vi "PropertyObjectFile Ref.vi"(8 "error in (no error)":errorcluster, 11 "PropertyObjectFile in":refnum<class "PropertyObjectFile.lvclass">) -> (0 "error out":errorcluster, 2 "PropertyObjectFile":refnum<k7>, 3 "PropertyObjectFile out":refnum<class "PropertyObjectFile.lvclass">)   [LabVIEW 2020, in "TSnax.lvlib" / "PropertyObjectFile.lvclass"]
uses:
  PropertyObjectFile.lvclass
  PropertyObjectFile.lvclass/PropertyObjectFile.ctl
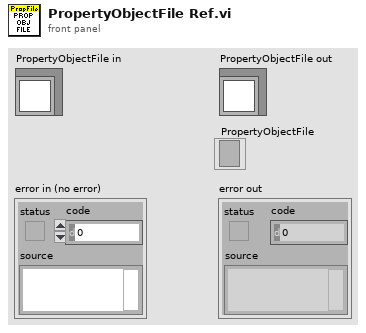
[diagram p1: front panel]
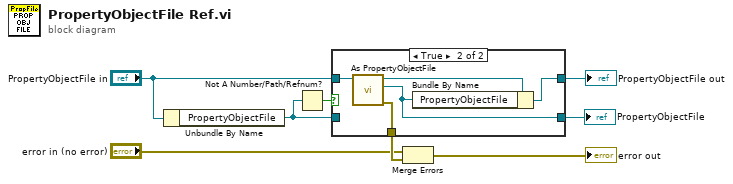
[diagram p0: block diagram]
diagram:
  n1 = Unbundle By Name("PropertyObjectFile in") -> ("PropertyObjectFile"=w5:refnum<k7>)
  n2 = Not A Number/Path/Refnum?(number/path/refnum=w5) -> (NaN/Path/Refnum?=w8:bool)
  n3 = case shown="True" w8 {
    tunnel: w5 -> [w9 _]
    tunnel: "PropertyObjectFile in" -> [w10 w15]
    tunnel: [w10 w13] -> w3
    tunnel: [_ w12] -> w7
    tunnel: [w9 w11] -> w4
    frame False {
    }
    frame True {
      n4 = call-dynamic "As PropertyObjectFile.vi"("PropertyObjectFile in"=w15) -> ("error out"=w12:errorcluster, "PropertyObjectFile"=w11:refnum<k7>, "PropertyObjectFile out"=w14:refnum<class "PropertyObjectFile.lvclass">)  [unwired: 8 in]
      n5 = Bundle By Name(cluster=w14, "PropertyObjectFile"=w11) -> (w13:refnum<class "PropertyObjectFile.lvclass">)
    }
  }
  "PropertyObjectFile out" <- w3
  "PropertyObjectFile" <- w4
  n6 = Merge Errors("error in (no error)", w7) -> (→"error out":errorcluster)
